vi "sort by unit id.vi"(11 "Channels":T1[](array[typedef])=[{"Name"="1", "Modbus Type"=enum."Coil", "Veristand Type"=enum."Input", "Mapping"={"DataType"=enum."Double", "Unit ID"=0, "Starting Address"=0, "Sub-Index (Bool)"=0, "VS Reference"=0}}, {"Name"="2", "Modbus Type"=enum."Coil", "Veristand Type"=enum."Input", "Mapping"={"DataType"=enum."Double", "Unit ID"=1, "Starting Address"=0, "Sub-Index (Bool)"=0, "VS Reference"=0}}, {"Name"="3", "Modbus Type"=enum."Coil", "Veristand Type"=enum."Input", "Mapping"={"DataType"=enum."Double", "Unit ID"=0, "Starting Address"=2, "Sub-Index (Bool)"=0, "VS Reference"=0}}, {"Name"="4", "Modbus Type"=enum."Coil", "Veristand Type"=enum."Input", "Mapping"={"DataType"=enum."Double", "Unit ID"=1, "Starting Address"=4, "Sub-Index (Bool)"=0, "VS Reference"=0}}] {"Mapping"."VS Reference" format="%.0x"}) -> (3 "Sorted Channels":T1[][](array[typedef]) {"Mapping"."VS Reference" format="%.0x"})   [LabVIEW 2021, in "Modbus Master System Explorer.lvlib"]
uses:
  Modbus Master System Explorer.lvlib
  Shared/Controls/Data Model/Channel.ctl
  Modbus Type.ctl
  <vilib>/NI VeriStand/Custom Device API/Custom Device Channel Type.ctl
  Shared/Controls/Data Model/Mapping.ctl
  Shared/Controls/Data Model/DataType.ctl
  <vilib>/NI VeriStand/Custom Device API/Custom Device Item Ref.ctl
  Shared/Modbus Master Shared.lvlib
  <vilib>/NI VeriStand/Custom Device API/Custom Device API.lvlib
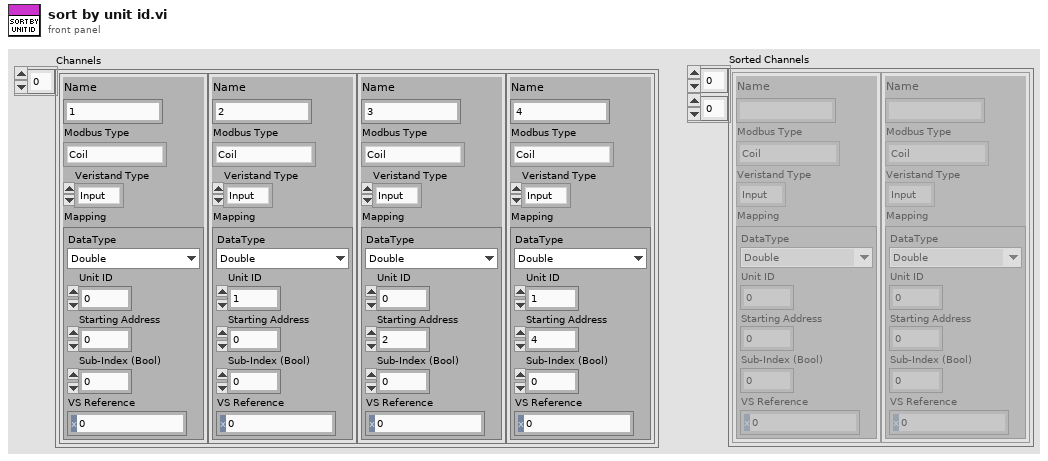
[diagram p1: front panel]
types:
  T1 = typedef "Modbus Master Shared.lvlib/Channel.ctl" = cluster{"Name":string, "Modbus Type":T2, "Veristand Type":T3, "Mapping":T4}
  T2 = typedef "Modbus Master Shared.lvlib/Modbus Type.ctl" = enum16{"Coil", "Discrete Input", "Holding Register", "Input Register"}
  T3 = typedef "Custom Device API.lvlib/Custom Device Channel Type.ctl" = enum16{"Input", "Output"}
  T4 = typedef "Modbus Master Shared.lvlib/Mapping.ctl" = cluster{"DataType":T5, "Unit ID":u8, "Starting Address":u16, "Sub-Index (Bool)":u16, "VS Reference":T6}
  T5 = typedef "Modbus Master Shared.lvlib/DataType.ctl" = enum16{"Double", "Single", "I64", "I32", "I16", "I8", "U64", "U32", "U16", "U8", "Boolean"}
  T6 = typedef "Custom Device API.lvlib/Custom Device Item Ref.ctl" = u64
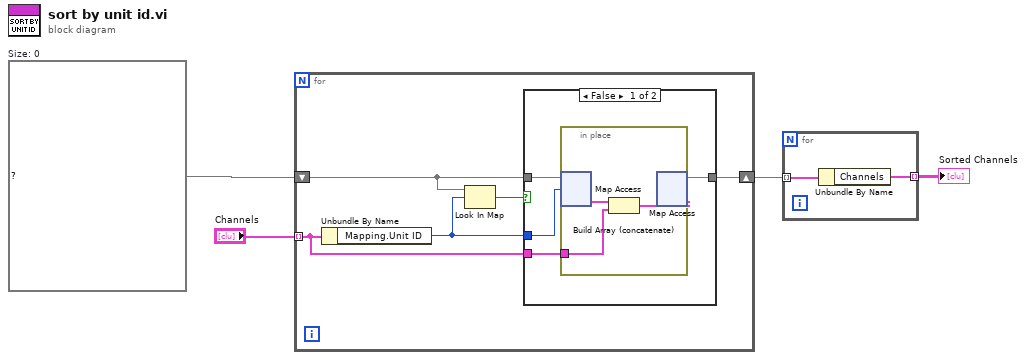
[diagram p0: block diagram]
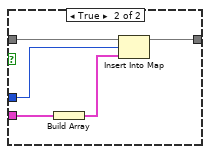
[diagram p2: hidden frame]
diagram:
  w3 = map{u8, T1[]} {}  # Size: 0
  n1 = for {
    tunnel: "Channels" -> [w6] mode=indexing
    shift-right: [w7] -> w2
    shift-left: w3 -> [w8]
    n2 = Unbundle By Name(w6) -> ("Mapping.Unit ID"=w5:u8)
    n3 = Look In Map(map=w8, key=w5) -> (key not found?=w9:bool)  [unwired: 1 in, 1 out]
    n4 = case shown="False" w9 {
      tunnel: w8 -> [w13 w21]
      tunnel: [w11 w20] -> w7
      tunnel: w6 -> [w10 w19]
      tunnel: w5 -> [w12 w18]
      frame False {
        n5 = in-place {
          in-place-border: w10 -> [w15]
          n6 = in-place-map #1(w13, w12) -> (w16:T1[])  [unwired: 1 in, 1 out]
          n7 = Build Array (concatenate)(w16, w15) -> (w14:T1[])
          n8 = in-place-map #1(w14) -> (w11:map{u8, T1[]})  [unwired: 1 in, 2 out]
        }
      }
      frame True {
        n9 = Build Array(w19) -> (w17:T1[])
        n10 = Insert Into Map(map in=w21, key=w18, value=w17) -> (map out=w20:map{u8, T1[]})  [unwired: 2 out]
      }
    }
  }
  n11 = for {
    tunnel: w2 -> [w23] mode=indexing
    tunnel: [w22] -> w1 mode=indexing
    n12 = Unbundle By Name(w23) -> ("Channels"=w22:T1[])
  }
  "Sorted Channels" <- w1
